vi "Channels Add.vi"(6 "WindowNumber":i32=1 format="%.0g", 7 "ChannelNumber":i32=1 format="%.0g", 8 "error in (no error)":errorcluster {"code" format="%.0x"}, 9 "ChannelParameter":string, 10 "ChannelType":string, 11 "instrument handle":refnum<k15>) -> (0 "error out":errorcluster {"code" format="%.0x"}, 2 "Val":i32, 3 "instrument handle out":refnum<k15>)   [LabVIEW 2014, in "Agilent NA.lvlib"]
doc: "Create particular measurement on a choosing channel and window."
uses:
  Agilent NA.lvlib
  AgNA.dll
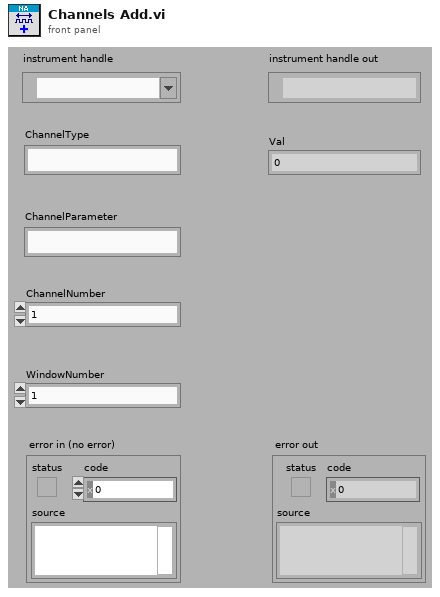
[diagram p1: front panel]
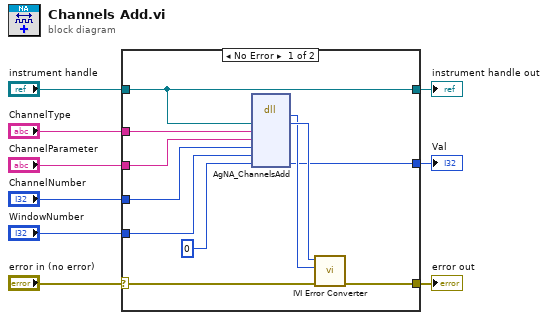
[diagram p0: block diagram]
diagram:
  n1 = case shown="No Error" "error in (no error)" {
    selector: "error in (no error)" -> [w18 w22]
    tunnel: [w17 w22] -> w9
    tunnel: "ChannelType" -> [w16 _]
    tunnel: "ChannelParameter" -> [w15 _]
    tunnel: "ChannelNumber" -> [w14 _]
    tunnel: "WindowNumber" -> [w13 _]
    tunnel: [w11 _] -> w3
    tunnel: [w10 w21] -> w2
    tunnel: "instrument handle" -> [w10 w21]
    frame No Error {
      n2 = dll-call lib="AgNA**.dll" fn="AgNA_ChannelsAdd"("Vi"=w10, "ChannelType"=w16, "ChannelParameter"=w15, "ChannelNumber"=w14, "WindowNumber"=w13, "Val"=0) -> (w19:i32, "Vi"=w20:u32, "Val"=w11:i32)  [unwired: 7 in, 2 out]
      n3 = call "IVI Error Converter.vi"("error in (no error)"=w18, "IVI error code (0)"=w19, "instrument handle"=w20) -> ("error out"=w17:errorcluster)  [unwired: 7 in, 1 out]
    }
    frame Error {
    }
  }
  "error out" <- w9
  "instrument handle out" <- w2
  "Val" <- w3
